vi "Switch Wait for Debounce.vi"(8 "error in (no error)":errorcluster, 11 "Switch Refs":refnum<k15>[](array[refnum])) -> (0 "error out":errorcluster)   [LabVIEW 2019]
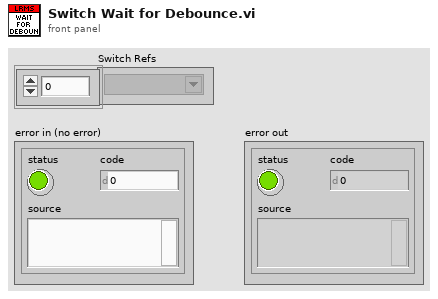
[diagram p1: front panel]
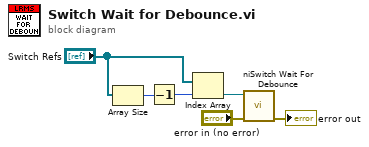
[diagram p0: block diagram]
diagram:
  n1 = Array Size(array="Switch Refs") -> (size(s)=w2:i32)
  n2 = Decrement(x=w2) -> (x-1=w3:i32)
  n3 = Index Array(array="Switch Refs", index=w3) -> (element=w4:refnum<k15>)
  n4 = call <instrlib>:"niSwitch Wait For Debounce.vi"("error in (no error)"="error in (no error)", "instrument handle"=w4) -> ("error out"=→"error out":errorcluster)  [unwired: 8 in, 1 out]
